vi "Step1.vi"() -> ()   [LabVIEW 2025]
uses:
  <vilib>/Utility/file.llb/Read Delimited Spreadsheet (DBL).vi
  <vilib>/Analysis/NI_AALBase.lvlib
panel:
  out "After Outlier Removal":waveform(dbl)(graph)
  in  "Z Threshold":dbl
  in  "Data File Path":path
  out "Time vs Signal":waveform(dbl)(graph)
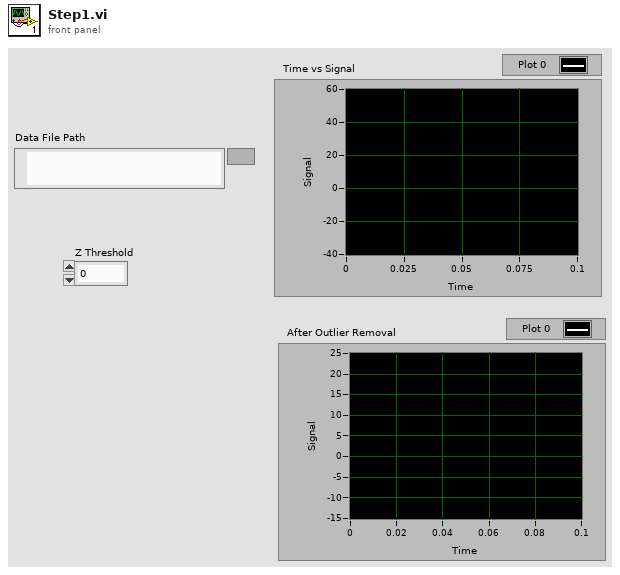
[diagram p1: front panel]
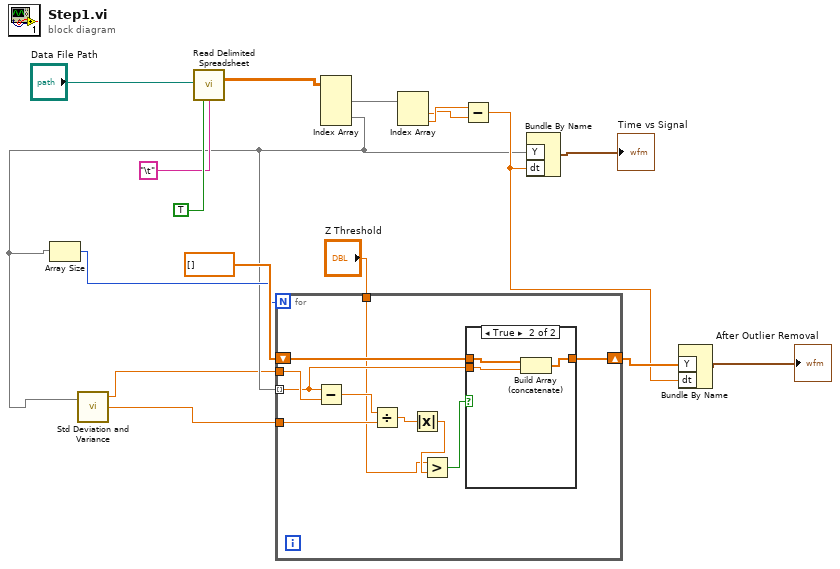
[diagram p0: block diagram]
diagram:
  n1 = call-poly <vilib>:"Read Delimited Spreadsheet.vi"("file path (dialog if empty)"="Data File Path", "transpose? (F)"=TRUE, "delimiter (\\t)"="\t" ("delimiter (\\t)")) -> ("all rows"=w15:dbl[][])  [unwired: 7 in, 5 out]
  n2 = Index Array(array=w15) -> (element #1=w14:dbl[], element #2=w3:dbl[])  [unwired: 4 in]
  n3 = Array Size(array=w3) -> (size(s)=w4:i32)
  n4 = call <vilib>:"Std Deviation and Variance.vi"("X"=w3) -> ("mean"=w2:dbl, "standard deviation"=w1:dbl)  [unwired: 1 in, 1 out]
  n5 = for {
    N: w4 -> [_]
    shift-right: [w20] -> w7
    shift-left: dbl[] [] -> [w21]
    tunnel: w1 -> [w26]
    tunnel: w3 -> [w22] mode=indexing
    tunnel: w2 -> [w24]
    tunnel: "Z Threshold" -> [w18]
    n6 = Subtract(x=w22, y=w24) -> (x-y=w27:dbl)
    n7 = Divide(x=w27, y=w26) -> (x/y=w25:dbl)
    n8 = Absolute Value(x=w25) -> (abs(x)=w19:dbl)
    n9 = Greater?(x=w18, y=w19) -> (0:w23:bool)
    n10 = case shown="True" w23 {
      tunnel: w22 -> [_ w30]
      tunnel: w21 -> [w28 w31]
      tunnel: [w28 w29] -> w20
      frame False {
      }
      frame True {
        n11 = Build Array (concatenate)(w31, w30) -> (w29:dbl[])
      }
    }
  }
  n12 = Index Array(array=w14) -> (element #1=w12:dbl, element #2=w13:dbl)  [unwired: 2 in]
  n13 = Subtract(x=w13, y=w12) -> (x-y=w5:dbl)
  n14 = Bundle By Name("Y"=w3, "dt"=w5) -> (→"Time vs Signal":waveform(dbl))  [unwired: 1 in]
  n15 = Bundle By Name("Y"=w7, "dt"=w5) -> (→"After Outlier Removal":waveform(dbl))  [unwired: 1 in]
